vi "AH2500_Queue_Commands.vi"(1 "AH2500-Control":T1, 3 "AH2500 Queue":refnum<queue> caption="5T Queue") -> (0 "New Status":T1)   [LabVIEW 2019]
uses:
  AH2500/AH2500-Control.ctl
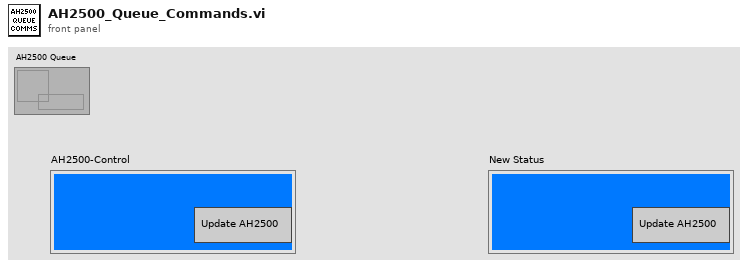
[diagram p1: front panel]
types:
  T1 = typedef "AH2500-Control.ctl" = cluster{"Update AH2500":bool}
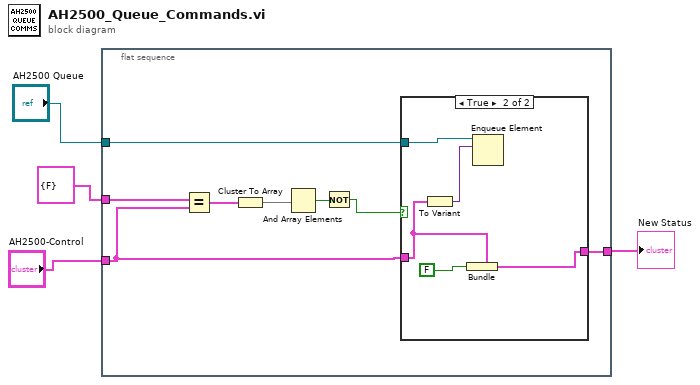
[diagram p0: block diagram]
diagram:
  n1 = flat-sequence {
    tunnel: T1 {"Update AH2500"=FALSE} ("AH2500-Control") -> [w12]
    tunnel: "AH2500-Control" -> [w7]
    tunnel: [w6] -> w2
    tunnel: "AH2500 Queue" -> [w5]
    frame #0 {
      n2 = Equal?(x=w12, y=w7) -> (x = y?=w11:T1)
      n3 = Cluster To Array(cluster=w11) -> (array=w10:bool[])
      n4 = And Array Elements(Boolean array=w10) -> (logical AND=w9:bool)
      n5 = Not(x=w9) -> (.not. x?=w8:bool)
      n6 = case shown="True" w8 {
        tunnel: w7 -> [w13 w16]
        tunnel: [w13 w14] -> w6
        tunnel: w5 -> [_ w18]
        frame False {
        }
        frame True {
          n7 = To Variant(anything=w16) -> (Variant=w17:variant)
          n8 = Bundle(cluster=w16, "Update AH2500"=FALSE) -> (w14:T1)
          n9 = Enqueue Element(queue=w18, element=w17) -> ()  [unwired: 2 in, 3 out]
        }
      }
    }
  }
  "New Status" <- w2
